vi "1 Nano Structure with 1 CNTs.vi"(0 "Radius of CNTs":dbl, 1 "m-nm r":dbl, 2 "Length of CNTs":dbl, 3 "m-nm l":dbl, 4 "Width of Base":dbl, 6 "m-nm Gap":dbl, 7 "m-nm WB":dbl, 8 "Gap Between CNTs":dbl, 9 "Length of Base":dbl, 11 "m-nm NS Base":dbl caption="m-nm 4") -> (5 "Length of CNTs":dbl, 10 "Area 1 CNT & Gap":dbl, 12 "CNT Radius":dbl, 13 "NS Length":dbl, 14 "CNT Base Area":dbl, 15 "Surface Area of 1 CNT":dbl, 16 "Surface Area 1 NS":dbl, 17 "# of CNTs in 1 NS":dbl, 18 "NS Base Area":dbl, 19 "NS Width":dbl)   [LabVIEW 2020]
panel:
  # "1 CNT"
  # "1 NanoStructure"
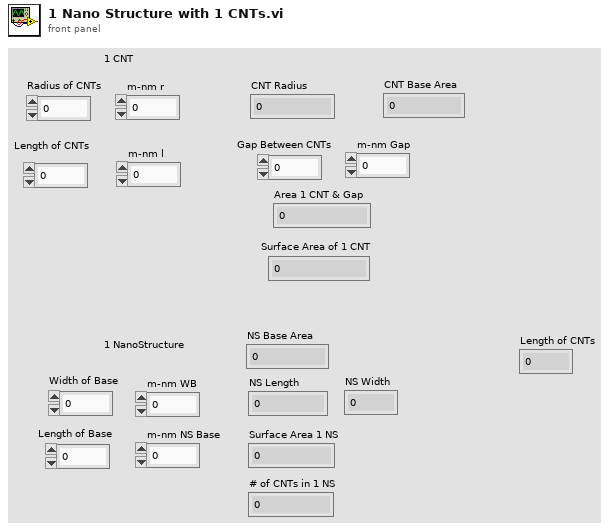
[diagram p1: front panel]
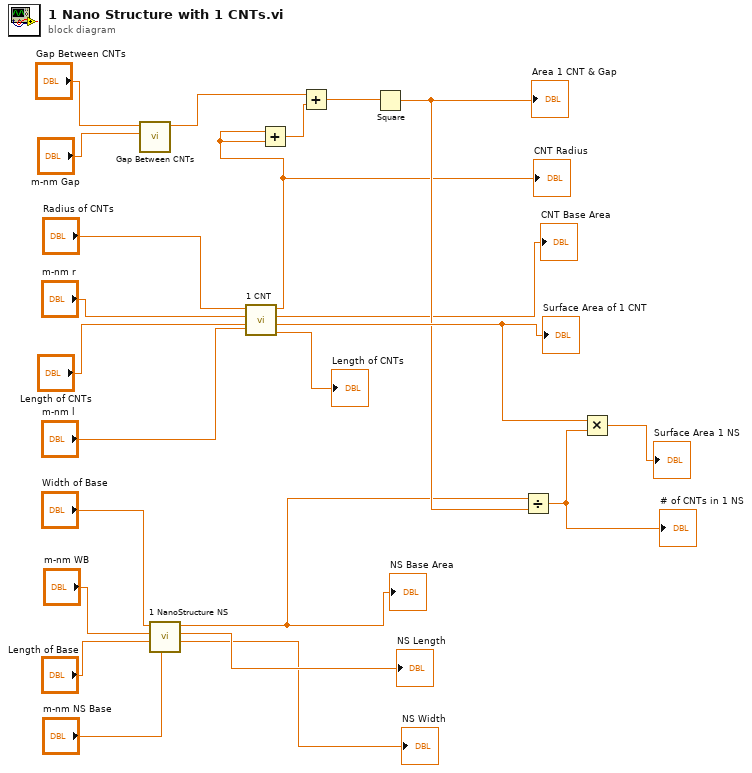
[diagram p0: block diagram]
diagram:
  n1 = call "Gap Between CNTs.vi"("m-nm Gap"="m-nm Gap", "Gap Between CNTs"="Gap Between CNTs") -> ("Numeric"=w10:dbl)  [unwired: 9 in]
  n2 = call "1 NanoStructure NS.vi"("m-nm 4"="m-nm NS Base", "Length of Base"="Length of Base", "m-nm WB"="m-nm WB", "Width of Base"="Width of Base") -> ("NS Width"=→"NS Width":dbl, "NS Length"=→"NS Length":dbl, "NS Base Area"=w20:dbl)  [unwired: 5 in]
  "NS Base Area" <- w20
  n3 = call "1 CNT.vi"("m-nm l"="m-nm l", "Length of CNTs"="Length of CNTs", "m-nm r"="m-nm r", "Radius of CNTs"="Radius of CNTs") -> ("Length of CNTs"=→"Length of CNTs":dbl, "Surface Area of 1 CNT"=w22:dbl, "CNT Base Area"=→"CNT Base Area":dbl, "CNT Radius"=w7:dbl)  [unwired: 4 in]
  "Surface Area of 1 CNT" <- w22
  "CNT Radius" <- w7
  n4 = Add(x=w7, y=w7) -> (x+y=w11:dbl)
  n5 = Add(x=w10, y=w11) -> (x+y=w12:dbl)
  n6 = Square(x=w12) -> (x^2=w21:dbl)
  "Area 1 CNT & Gap" <- w21
  n7 = Divide(x=w20, y=w21) -> (x/y=w17:dbl)
  "# of CNTs in 1 NS" <- w17
  n8 = Multiply(x=w22, y=w17) -> (x*y=→"Surface Area 1 NS":dbl)
